vi "Add Build.vi"(6 "Project Path":path, 7 "Build Object type":T1, 8 "error in (no error)":errorcluster, 9 "Build Specification":string, 10 "Target Name":string, 11 "Builder in":refnum<class "Builder.lvclass">) -> (0 "error out":errorcluster, 3 "Builder out":refnum<class "Builder.lvclass">)   [LabVIEW 2025, in "App-Builder Library.lvlib" / "Builder.lvclass"]
uses:
  Builder.lvclass
  Build object type.ctl
  Builder.lvclass/Builder.ctl
  Build specification.ctl
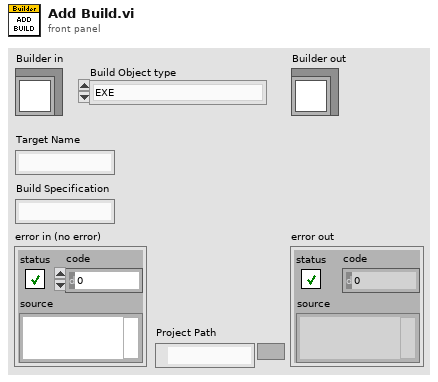
[diagram p1: front panel]
types:
  T1 = typedef "App-Builder Library.lvlib/Builder.lvclass/Build object type.ctl" = enum16{"EXE", "RT EXE", "Deployable Packed"}
  T2 = typedef "App-Builder Library.lvlib/Builder.lvclass/Build specification.ctl" = cluster{"target name":string, "Build specification":string, "Project Path":path, "Build Object type":T1}
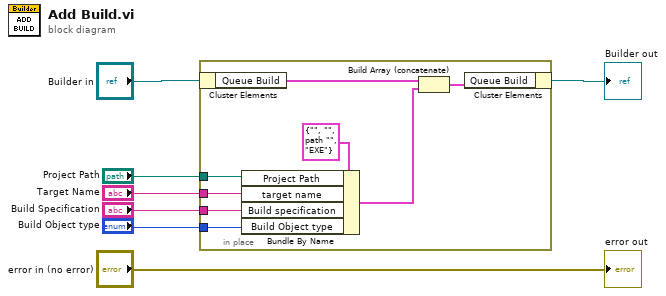
[diagram p0: block diagram]
diagram:
  n1 = in-place {
    in-place-border: "Project Path" -> [w15]
    in-place-border: "Target Name" -> [w14]
    in-place-border: "Build Specification" -> [w13]
    in-place-border: "Build Object type" -> [w8]
    n2 = in-place-cluster #1("Builder in") -> ("Queue Build"=w12:T2[])
    n3 = Bundle By Name(cluster=T2 {"target name"="", "Build specification"="", "Project Path"=path "", "Build Object type"=enum."EXE"} ("Queue Build"), "Project Path"=w15, "target name"=w14, "Build specification"=w13, "Build Object type"=w8) -> (w9:T2)
    n4 = Build Array (concatenate)(w12, w9) -> (w11:T2[])
    n5 = in-place-cluster #1("Queue Build"=w11) -> (→"Builder out":refnum<class "Builder.lvclass">)
  }
  "error out" <- "error in (no error)"
